vi "GetWindowSurfaceVSync.vi"(8 "No Error":errorcluster, 11 "Window [SDL_Window *]":i64 format="%.0x") -> (0 "Error Out":errorcluster, 2 "Window Surface VSync":T1 items=["SDL_WINDOW_SURFACE_VSYNC_DISABLED"=0, "SDL_WINDOW_SURFACE_VSYNC_ADAPTIVE"=-1], 3 "Surface [SDL_Surface *]":i64 format="%.0x")   [LabVIEW 2024, in "SDL3.lvlib" / "Video.lvlib"]
doc: "<B>Summary</B>\nGet VSync for the window surface.\n\n<B>Remarks</B>\nWindow Surface VSync can be more than 0 or -1"
uses:
  Video.lvlib
  WindowSurfaceVSync--ring.ctl
  Error/Error.lvlib
  Lib/SDL3-32.dll
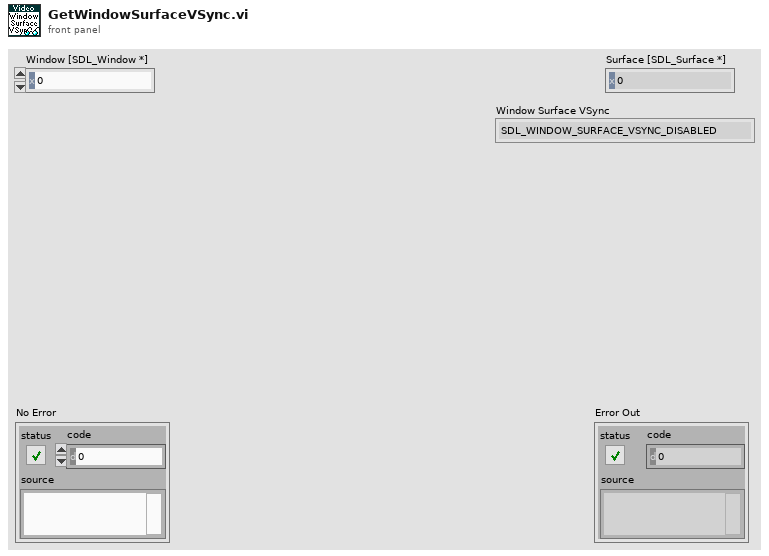
[diagram p1: front panel]
types:
  T1 = typedef "SDL3.lvlib/Video.lvlib/WindowSurfaceVSync--ring.ctl" = i32
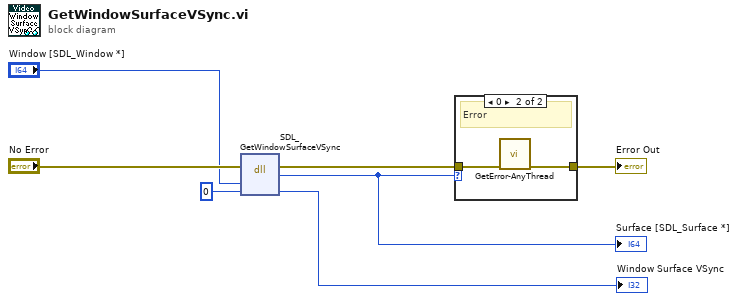
[diagram p0: block diagram]
diagram:
  n1 = dll-call lib="C:/Users/Thomas/Documents/Projects/LV-SDL3/Lib/SDL3-*.*" fn="SDL_GetWindowSurfaceVSync"(error in="No Error", "window"="Window [SDL_Window *]", "vsync"=0) -> (error out=w4:errorcluster, "return type"=w3:i64, "vsync"=→"Window Surface VSync":i32)  [unwired: 3 in, 1 out]
  "Surface [SDL_Surface *]" <- w3
  n2 = case shown="0" w3 {
    tunnel: w4 -> [w8 w10]
    tunnel: [w8 w9] -> w6
    frame Default {
      # "Ok"
    }
    frame 0 {
      # "Error"
      n3 = call "GetError-AnyThread.vi"("No Error"=w10) -> ("Error Out"=w9:errorcluster)  [unwired: 10 in]
    }
  }
  "Error Out" <- w6
